vi "Actor Core.vi"(8 "error in":errorcluster, 11 "Error Display Actor In":refnum<class "Error Display Actor.lvclass">) -> (0 "error out":errorcluster, 3 "Actor out":refnum<class "Actor.lvclass">)   [LabVIEW 2020, in "ViewableActor.lvlib" / "Error Display Actor.lvclass"]
uses:
  Error Display Actor.lvclass
  C:/Users/AlexK/work/LabVIEW Programme/POLARIS CAM Log Abw und E/Submodules/Viewable Actor/ViewableActor/ViewableActor.lvclass
  C:/Program Files (x86)/National Instruments/LabVIEW 2020/vi.lib/ActorFramework/Actor/Actor.lvclass
  <vilib>/ActorFramework/Actor/Actor.lvclass
  Error Display Actor.lvclass/Error Display Actor.ctl
  ViewableActor/ViewableActor.lvclass/ViewableActor.ctl
  <vilib>/ActorFramework/Actor/Actor.lvclass/Actor.ctl
  <vilib>/ActorFramework/Message Enqueuer/Message Enqueuer.lvclass/Message Enqueuer.ctl
  Read Source Actor.vi
  Read error for msg.vi
  ViewableActor/Read Stop Event.vi
  <vilib>/ActorFramework/Message Enqueuer/Init from Existing Queue.vi
  <vilib>/ActorFramework/Message Enqueuer/Enqueue.vi
  <vilib>/ActorFramework/Stop Msg/Stop Msg.lvclass
  C:/Program Files (x86)/National Instruments/LabVIEW 2020/vi.lib/ActorFramework/Message/Message.lvclass
  <vilib>/ActorFramework/Message Priority Queue/Priority Enqueue.vi
  <vilib>/ActorFramework/Message Enqueuer/Message Enqueuer.lvclass
  ViewableActor/ViewableActor.lvclass
panel:
  out "Actor":string
  out "error for msg":errorcluster
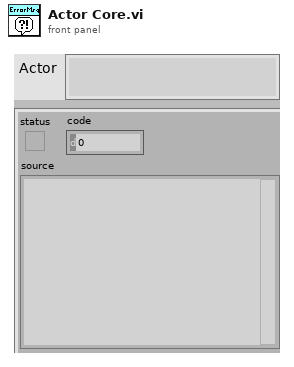
[diagram p1: front panel]
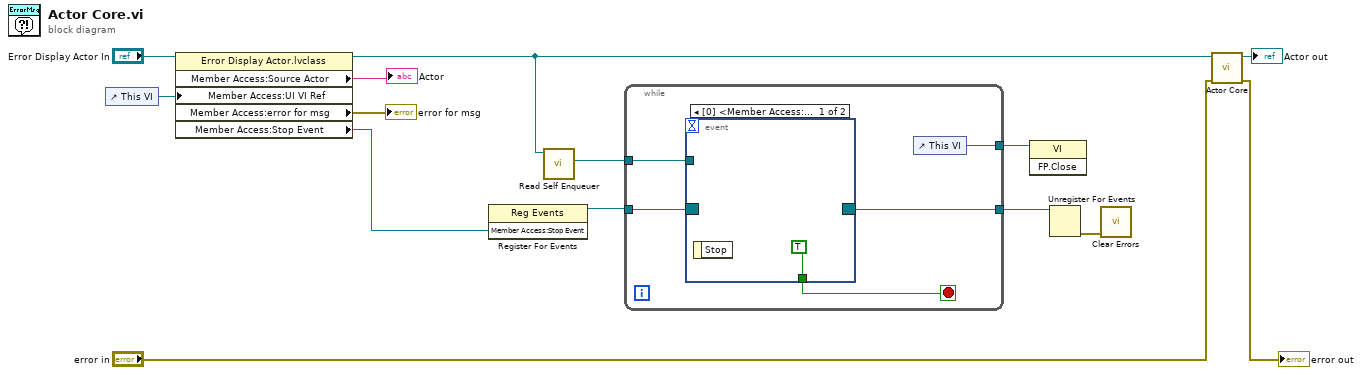
[diagram p0: block diagram]
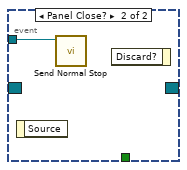
[diagram p2: hidden frame]
diagram:
  n1 = control-ref of="This VI"() -> (w10:refnum<vi>)
  n2 = property class="Error Display Actor.lvclass"(reference="Error Display Actor In", "Member Access:UI VI Ref"=w10) -> (reference out=w5:refnum<class "Error Display Actor.lvclass">, "Member Access:Source Actor"=→"Actor":string, "Member Access:error for msg"=→"error for msg":errorcluster, "Member Access:Stop Event"=w8:refnum<user-event>)  [unwired: 1 in, 1 out]
  n3 = register-events(w8) -> (reference out=w7:refnum<event-registration>)  [unwired: 2 in, 1 out]
  n4 = call <vilib>:"Read Self Enqueuer.vi"("Actor"=w5) -> ("Self Enqueuer"=w4:refnum<class "Message Enqueuer.lvclass">)  [unwired: 10 in]
  n5 = while {
    tunnel: w7 -> [w19]
    tunnel: w4 -> [w17]
    tunnel: [w16] -> w3
    tunnel: [w15] -> w1
    stop <- w18 stop-if-true
    n6 = event shown="[0] <Member Access:Stop Event>: User Event" {
      selector: w19 -> [_ _]
      dyn-events: [_ _] -> w16
      timeout: _ -> [_ _]
      tunnel: [TRUE _] -> w18
      tunnel: w17 -> [_ w21]
      event User Event {
        n7 = event-data() -> ()  [unwired: 1 in, 1 out]
      }
      event Panel Close? {
        n8 = event-data() -> ()  [unwired: 1 in, 1 out]
        n9 = call <vilib>:"Send Normal Stop.vi"("Message Enqueuer"=w21) -> ()  [unwired: 10 in, 1 out]
        n10 = event-data() -> ()  [unwired: 2 in, 1 out]
      }
    }
    n11 = control-ref of="This VI"() -> (w15:refnum<vi>)
  }
  n12 = invoke class="VI" method="FP.Close"(reference=w1) -> ()  [unwired: 2 in, 3 out]
  n13 = Unregister For Events(event registration refnum=w3) -> (error out=w2:errorcluster)  [unwired: 1 in]
  n14 = call <vilib>:"Clear Errors.vi"("error in (no error)"=w2) -> ()  [unwired: 5 in, 2 out]
  n15 = call-parent "Actor Core.vi"("error in"="error in", "Actor in"=w5) -> ("error out"=→"error out":errorcluster, "Actor out"=→"Actor out":refnum<class "Actor.lvclass">)  [unwired: 8 in]
